vi "GVAIs_ECD.vi"() -> ()   [LabVIEW 2017]
panel:
  in  "AIs":dbl[](array[numeric])
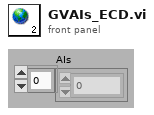
[diagram p1: front panel]
diagram:
